vi "CRYUnit Prefix to Multiplier.vi"(5 "unit prefix":string) -> (2 "multiplier":dbl=1.0 format="%.2e")   [LabVIEW 2013]
panel:
  in  "prefix-multiplier pairs":cluster{"prefix":string, "multiplier":dbl}[](array[cluster])=[{"prefix"="a", "multiplier"=1e-18}, {"prefix"="f", "multiplier"=1e-15}, {"prefix"="p", "multiplier"=1e-12}, {"prefix"="n", "multiplier"=1e-09}, {"prefix"="µ", "multiplier"=1e-06}, {"prefix"="u", "multiplier"=1e-06}, {"prefix"="m", "multiplier"=0.001}, {"prefix"="c", "multiplier"=0.01}, {"prefix"="da", "multiplier"=10.0}, {"prefix"="d", "multiplier"=0.1}, {"prefix"="h", "multiplier"=100.0}, {"prefix"="k", "multiplier"=1000.0}, {"prefix"="M", "multiplier"=1000000.0}, {"prefix"="G", "multiplier"=1000000000.0}, {"prefix"="T", "multiplier"=1000000000000.0}, {"prefix"="P", "multiplier"=1000000000000000.0}, {"prefix"="E", "multiplier"=1e+18}] {"multiplier" format="%.2e"}
  # "NOTE: micro is denoted\n  either by \"u\" or by \"m \",\n  m with a space after it"
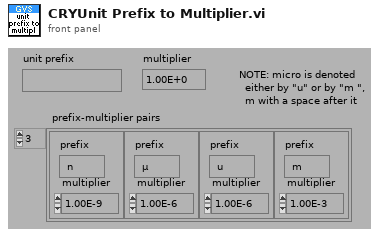
[diagram p1: front panel]
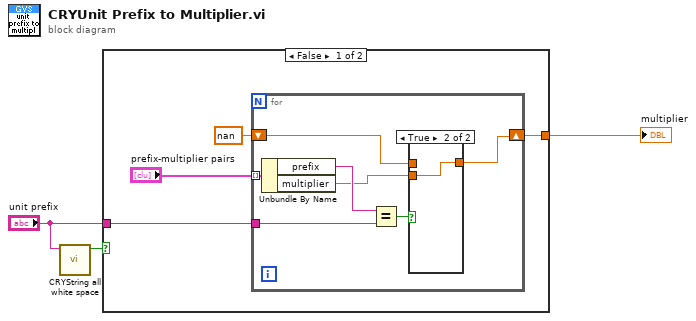
[diagram p0: block diagram]
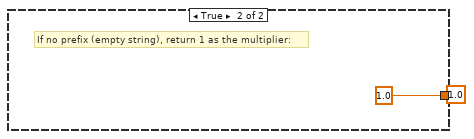
[diagram p3: hidden frame]
diagram:
  n1 = call "CRYString all white space.vi"("String"="unit prefix") -> ("Nothing but white space?"=w2:bool)  [unwired: 10 out]
  n2 = case shown="False" w2 {
    tunnel: "unit prefix" -> [w6 _]
    tunnel: [w4 1.0 ("multiplier")] -> w1
    frame False {
      n3 = for {
        tunnel: "prefix-multiplier pairs" -> [w14] mode=indexing
        tunnel: w6 -> [w9]
        shift-right: [w10] -> w4
        shift-left: nan -> [w12]
        n4 = Unbundle By Name(w14) -> ("prefix"=w13:string, "multiplier"=w11:dbl)
        n5 = Equal?(x=w13, y=w9) -> (x = y?=w8:bool)
        n6 = case shown="True" w8 {
          tunnel: w12 -> [w15 _]
          tunnel: w11 -> [_ w16]
          tunnel: [w15 w16] -> w10
          frame False {
          }
          frame True {
          }
        }
      }
    }
    frame True {
      (unwired) 1.0
      # "If no prefix (empty string), return 1 as the multiplier:"
    }
  }
  "multiplier" <- w1
